vi "Read Valve Position.vi"(8 "error in (no error)":errorcluster, 11 "Valve in":refnum<class "Valve.lvclass">) -> (0 "error out":errorcluster, 2 "Valve Position":refnum<vi>, 3 "Valve out":refnum<class "Valve.lvclass">)   [LabVIEW 2013, in "Valve.lvlib" / "Valve.lvclass"]
uses:
  Valve.lvclass
  Valve.lvclass/Valve.ctl
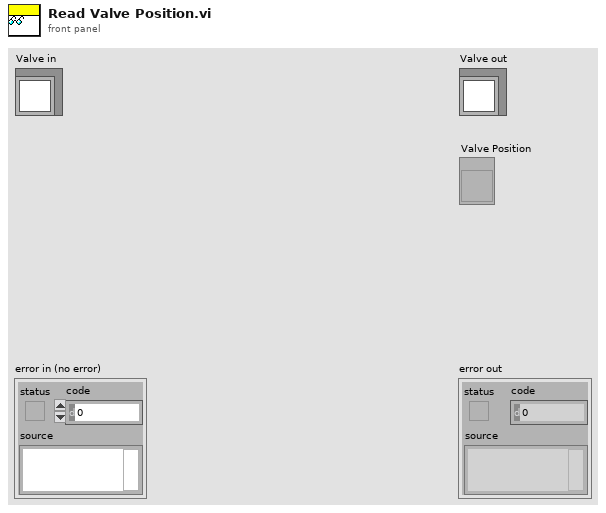
[diagram p1: front panel]
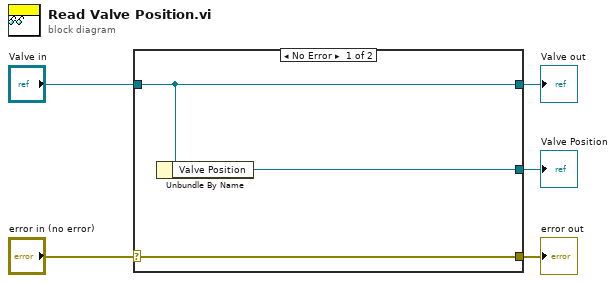
[diagram p0: block diagram]
diagram:
  n1 = case shown="No Error" "error in (no error)" {
    selector: "error in (no error)" -> [w8 w9]
    tunnel: [w8 w9] -> w4
    tunnel: [w7 w10] -> w2
    tunnel: "Valve in" -> [w7 w10]
    tunnel: [w6 _] -> w1
    frame No Error {
      n2 = Unbundle By Name(w7) -> ("Valve Position"=w6:refnum<vi>)
    }
    frame Error {
    }
  }
  "error out" <- w4
  "Valve out" <- w2
  "Valve Position" <- w1
